vi "PathPlanner_FieldUtil_FlipFeedforwards.vi"(11 "Feedforward":dbl[](array[numeric])) -> (3 "FlippedFeedforward":dbl[](array[numeric]))   [LabVIEW 2019, in "PathPlanner24.lvlib"]
doc: "Flip a field position\n\nInput:\n -- FieldPosition\n\nOutputs:\n -- FlippedFieldPosition"
uses:
  PathPlanner_FieldUtil_FieldSizeY.vi
  <vilib>/Rock Robotics/WPI/ThirdParty/JAS_Junk/TrajLib/Translation2d_GetXY.vi
  <vilib>/Rock Robotics/WPI/ThirdParty/JAS_Junk/TrajLib/Translation2d_Create.vi
  PathPlanner_FieldUtil_FieldSizeX.vi
  <vilib>/Rock Robotics/WPI/ThirdParty/JAS_Junk/TrajLib/Rotation2d_CreateAngle.vi
  <vilib>/Rock Robotics/WPI/ThirdParty/JAS_Junk/TrajLib/Rotation2d_Minus.vi
  <vilib>/Rock Robotics/WPI/ThirdParty/JAS_Junk/TrajLib/Conv_Feet_Meters.vi
  <vilib>/Rock Robotics/WPI/ThirdParty/JAS_Junk/TrajLib/Rotation2d_UnaryMinus.vi
  <vilib>/Rock Robotics/WPI/ThirdParty/JAS_Junk/TrajLib/Rotation2d_RotateBy.vi
  <vilib>/Rock Robotics/WPI/ThirdParty/JAS_Junk/TrajLib/Rotation2d_CreateXY.vi
  <vilib>/Rock Robotics/WPI/ThirdParty/JAS_Junk/TrajLib/Util_CalcDist.vi
  PathPlanner24.lvlib
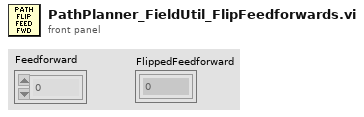
[diagram p1: front panel]
types:
  T1 = typedef "PathPlanner24.lvlib/PathPlanner_FieldSymmetry_ENUM.ctl" = enum16{"kRotational", "kMirrored"}
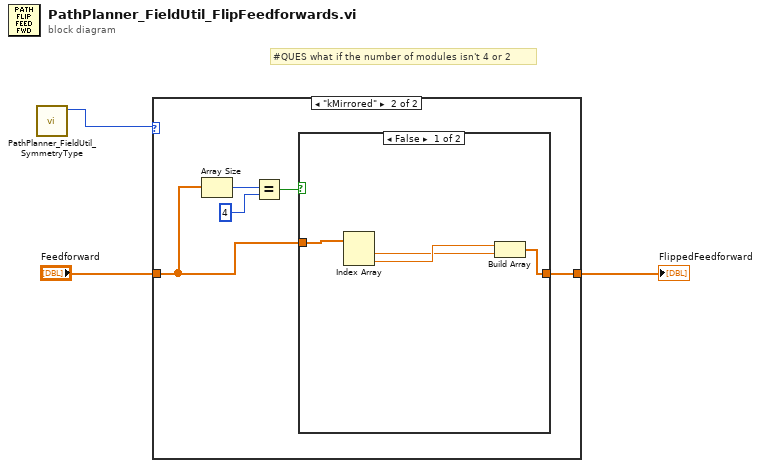
[diagram p0: block diagram]
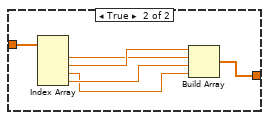
[diagram p3: hidden frame]
diagram:
  # "#QUES what if the number of modules isn't 4 or 2"
  n1 = call "PathPlanner_FieldUtil_SymmetryType.vi"() -> ("PathPlanner_FieldSymmetry"=w3:T1)  [unwired: 11 in]
  n2 = case shown="\"kMirrored\"" w3 {
    tunnel: "Feedforward" -> [w4 w6]
    tunnel: [w4 w5] -> w1
    frame "kRotational" {
    }
    frame "kMirrored" {
      n3 = Array Size(array=w6) -> (size(s)=w9:i32)
      n4 = Equal?(x=w9, y=4) -> (x = y?=w7:bool)
      n5 = case shown="False" w7 {
        tunnel: w6 -> [w11 w19]
        tunnel: [w10 w14] -> w5
        frame False {
          n6 = Index Array(array=w11) -> (element #1=w12:dbl, element #2=w13:dbl)  [unwired: 2 in]
          n7 = Build Array(w13, w12) -> (w10:dbl[])
        }
        frame True {
          n8 = Index Array(array=w19) -> (element #1=w17:dbl, element #2=w18:dbl, element #3=w15:dbl, element #4=w16:dbl)  [unwired: 4 in]
          n9 = Build Array(w18, w17, w16, w15) -> (w14:dbl[])
        }
      }
    }
  }
  "FlippedFeedforward" <- w1
